vi "Get NVMEM Bytes.vi"(0 "SLSC Interface In":refnum<class "SLSC Interface.lvclass">, 5 "NVMEM area":refnum<k21>="$DefaultNVMEMAreas", 7 "data address":u32 format="%.0x", 9 "data size":u32, 11 "error in (no error)":errorcluster) -> (4 "SLSC Interface Out":refnum<class "SLSC Interface.lvclass">, 6 "NVMEM area out":refnum<k21>, 8 "next data address":u32 format="%.0x", 10 "data out":u8[](array[numeric]) format="%.0x", 15 "error out":errorcluster)   [LabVIEW 2015, in "SLSC Interfaces.lvlib" / "SLSC Interface.lvclass"]
uses:
  SLSC Interface.lvclass
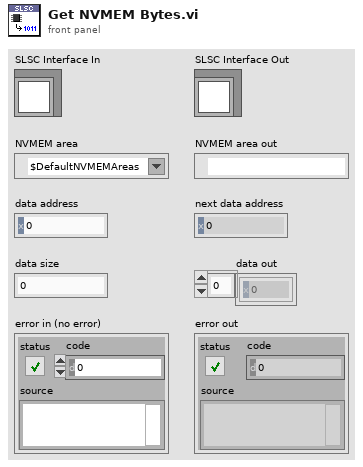
[diagram p1: front panel]
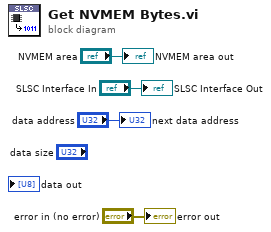
[diagram p0: block diagram]
diagram:
  "error out" <- "error in (no error)"
  "next data address" <- "data address"
  "NVMEM area out" <- "NVMEM area"
  "SLSC Interface Out" <- "SLSC Interface In"
